vi "Initialize Wfm Grp Ctrls.vi"(8 "error in (no error)":errorcluster, 11 "Ctrl Refs":T1) -> (0 "error out":errorcluster, 3 "To Save Wfm Arrays":waveform(dbl)[](array[waveform]))   [LabVIEW 2025, in "TDMS Waveform Creator UI.lvlib"]
uses:
  TDMS Waveform Creator UI.lvlib
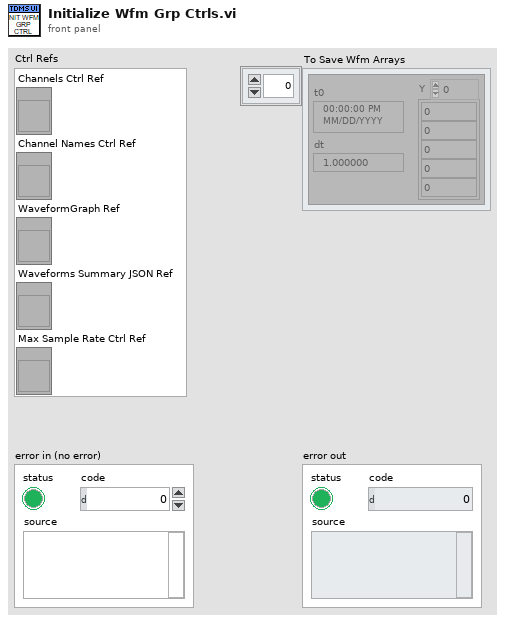
[diagram p1: front panel]
types:
  T1 = cluster{"Channels Ctrl Ref":refnum<vi>, "Channel Names Ctrl Ref":refnum<vi>, "WaveformGraph Ref":refnum<vi>, "Waveforms Summary JSON Ref":refnum<vi>, "Max Sample Rate Ctrl Ref":refnum<vi>}
  T2 = cluster{"Trim and Resample Settings":cluster{"Duration":dbl, "Sample Rate":dbl}, "Wfms Json":string[]}
  T3 = cluster{"File Path":string, "Sample Rate (Hz)":dbl, "Read From":i32, "Pre Delay (s)":dbl, "Post Delay (s)":dbl, "Scale":dbl}
  T4 = cluster{"Waveform Type":i32, "Sample Rate (Hz)":dbl, "Frequency (Hz)":dbl, "Amplitude":dbl, "Number of Cycles":u32, "Ramp Start":dbl, "Ramp Stop":dbl, "Length (s)":dbl, "DC Value":dbl, "Duration (s)":dbl, "Pre Delay (s)":dbl, "Post Delay (s)":dbl}
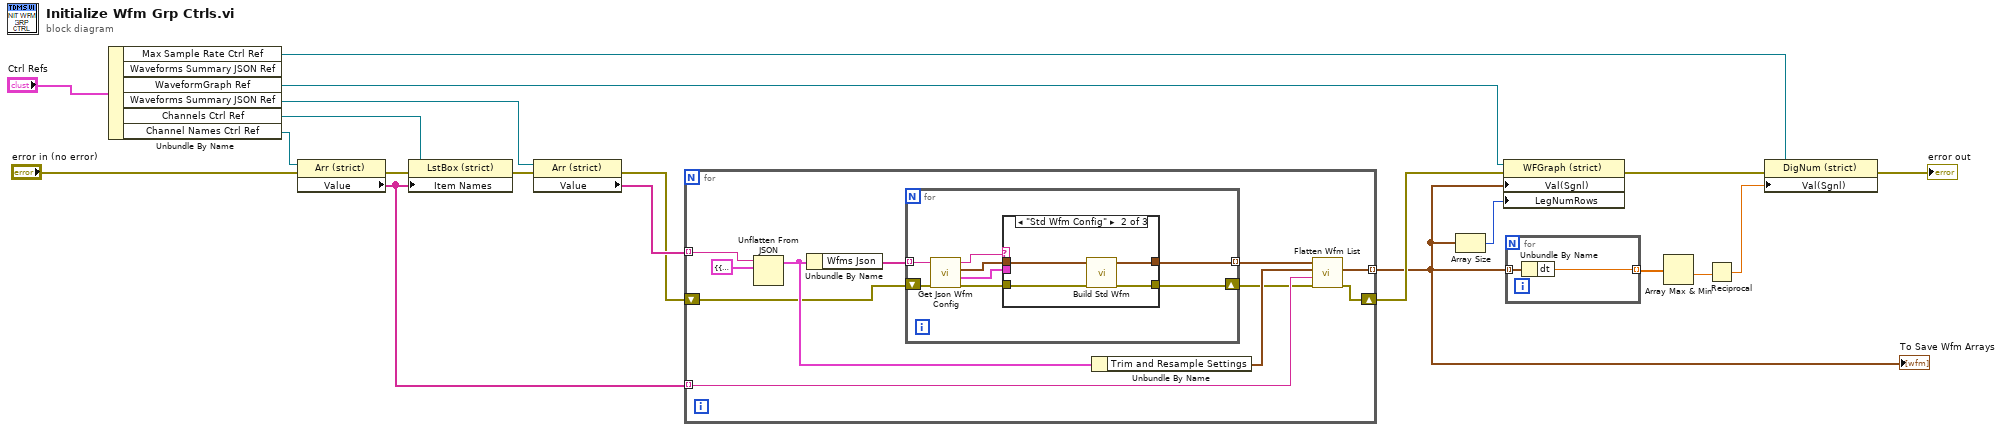
[diagram p0: block diagram]
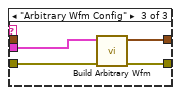
[diagram p3: hidden frame]
diagram:
  n1 = Unbundle By Name("Ctrl Refs") -> ("Max Sample Rate Ctrl Ref"=w12:refnum<vi>, "WaveformGraph Ref"=w15:refnum<vi>, "Waveforms Summary JSON Ref"=w8:refnum<vi>, "Channels Ctrl Ref"=w3:refnum<vi>, "Channel Names Ctrl Ref"=w16:refnum<vi>)  [unwired: 1 out]
  n2 = property on="Property Node" class="Arr (strict)"(reference=w16, error in="error in (no error)") -> (error out=w20:errorcluster, "Value"=w2:string[])  [unwired: 1 out]
  n3 = property class="LstBox (strict)"(reference=w3, error in=w20, "Item Names"=w2) -> (error out=w4:errorcluster)  [unwired: 1 out]
  n4 = property class="Arr (strict)"(reference=w8, error in=w4) -> (error out=w6:errorcluster, "Value"=w7:string[])  [unwired: 1 out]
  n5 = for {
    tunnel: w7 -> [w30] mode=indexing
    tunnel: w2 -> [w25] mode=indexing
    tunnel: [w23] -> w1 mode=indexing
    shift-right: [w21] -> w5
    shift-left: w6 -> [w22]
    n6 = Unflatten From JSON(JSON string=w30, type and defaults=T2 {"Trim and Resample Settings"={"Duration"=0.0, "Sample Rate"=0.0}, "Wfms Json"=[]} ("Wfm Summary")) -> (value=w27:T2)  [unwired: 5 in, 1 out]
    n7 = Unbundle By Name(w27) -> ("Wfms Json"=w29:string[])
    n8 = for {
      tunnel: w29 -> [w39] mode=indexing
      shift-right: [w34] -> w24
      shift-left: w22 -> [w33]
      tunnel: [w32] -> w28 mode=indexing
      n9 = call "Get Json Wfm Config.vi"("error in"=w33, "Json String"=w39) -> ("error out"=w36:errorcluster, "Arbitrary Wfm Config"=w35:T3, "Std Wfm Config"=w37:T4, "Type"=w38:string)  [unwired: 6 in]
      n10 = case shown="\"Std Wfm Config\"" w38 {
        tunnel: w37 -> [_ w41 _]
        tunnel: w36 -> [w40 w44 w48]
        tunnel: w35 -> [_ _ w47]
        tunnel: [_ w42 w46] -> w32
        tunnel: [w40 w43 w45] -> w34
        frame Default {
        }
        frame "Std Wfm Config" {
          n11 = call "Build Std Wfm.vi"("error in"=w44, "Standard Wfm Config"=w41) -> ("error out"=w43:errorcluster, "Waveform"=w42:waveform(dbl))  [unwired: 6 in, 2 out]
        }
        frame "Arbitrary Wfm Config" {
          n12 = call "Build Arbitrary Wfm.vi"("error in"=w48, "Arbitrary Wfm Config"=w47) -> ("error out"=w45:errorcluster, "Waveform"=w46:waveform(dbl))  [unwired: 6 in, 2 out]
        }
      }
    }
    n13 = Unbundle By Name(w27) -> ("Trim and Resample Settings"=w26:cluster{"Duration":dbl, "Sample Rate":dbl})
    n14 = call "Flatten Wfm List.vi"("error in (no error)"=w24, "Channel Name"=w25, "Trim and Resample Settings"=w26, "Canvas Wfm Array In"=w28) -> ("error out"=w21:errorcluster, "Final Flatten Wfm Channel"=w23:waveform(dbl))  [unwired: 5 in, 1 out]
  }
  "To Save Wfm Arrays" <- w1
  n15 = Array Size(array=w1) -> (size(s)=w18:i32)
  n16 = property on="Property Node" class="WFGraph (strict)"(reference=w15, error in=w5, "Val(Sgnl)"=w1, "LegNumRows"=w18) -> (error out=w14:errorcluster)  [unwired: 1 out]
  n17 = for {
    tunnel: [w50] -> w11 mode=indexing
    tunnel: w1 -> [w49] mode=indexing
    n18 = Unbundle By Name(w49) -> ("dt"=w50:dbl)
  }
  n19 = Array Max & Min(array=w11) -> (min value=w10:dbl)  [unwired: 3 out]
  n20 = Reciprocal(x=w10) -> (1/x=w9:dbl)
  n21 = property class="DigNum (strict)"(reference=w12, error in=w14, "Val(Sgnl)"=w9) -> (error out=→"error out":errorcluster)  [unwired: 1 out]
